vi "Is Empty.vi"(8 "error in (no error)":errorcluster) -> (0 "error out":errorcluster, 3 "Empty?":bool)   [LabVIEW 2022 SP3, in "hse-db.lvlib" / "DB_CONNECTOR.lvlib" / "Clone Registration.lvlib"]
doc: "Determine if the cloneable module registry is empty.\n____\nHAMPEL SOFTWARE ENGINEERING v1.4.0 (2023-12-19 09:52)"
uses:
  Clone Registration.lvlib
  Action--enum.ctl
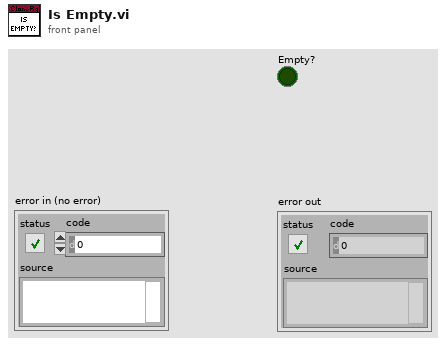
[diagram p1: front panel]
types:
  T1 = typedef "hse-db.lvlib/DB_CONNECTOR.lvlib/Clone Registration.lvlib/Action--enum.ctl" = enum16{"Init", "Add Instance", "Remove Instance", "List Instances", "Is First?"}
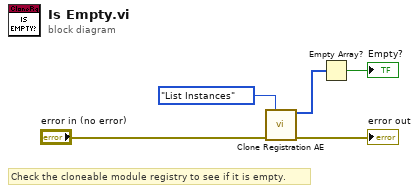
[diagram p0: block diagram]
diagram:
  # "Check the cloneable module registry to see if it is empty."
  n1 = call "Clone Registration AE.vi"("Action"=Action--enum."List Instances", "error in (no error)"="error in (no error)") -> ("Module IDs"=w1:i32[], "error out"=→"error out":errorcluster)  [unwired: 5 in, 7 out]
  n2 = Empty Array?(array=w1) -> (empty?=→"Empty?":bool)
